vi "PLC Queue Ref Holder.vi"(6 "Action":enum16{"GET", "SET"}(ring), 8 "error in":errorcluster, 11 "Message Queue In":refnum<queue>) -> (0 "error out":errorcluster, 3 "Input Message Queue":refnum<queue>)   [LabVIEW 2015, in "PLC.lvlib"]
uses:
  PLC.lvlib
  support/Message Queue/Message Cluster.ctl
  support/Message Queue/Message Queue.lvlib
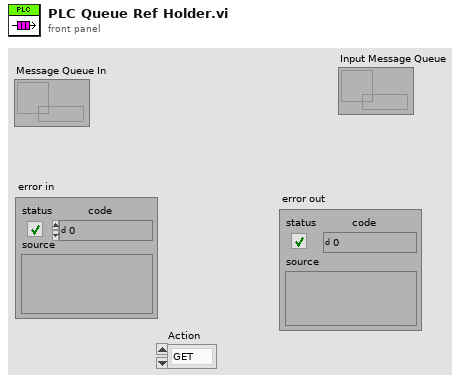
[diagram p1: front panel]
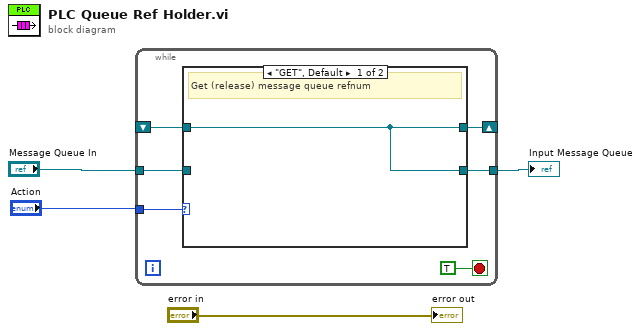
[diagram p0: block diagram]
diagram:
  n1 = while {
    shift-right: [w9] -> _
    shift-left: _ -> [w6]
    tunnel: "Message Queue In" -> [w8]
    tunnel: [w7] -> w3
    tunnel: "Action" -> [w5]
    stop <- TRUE stop-if-true
    n2 = case shown="\"GET\", Default" w5 {
      tunnel: [w11 w12] -> w9
      tunnel: w8 -> [_ w12]
      tunnel: [w11 w12] -> w7
      tunnel: w6 -> [w11 _]
      frame "GET", Default {
        # "Get (release) message queue refnum"
      }
      frame "SET" {
        # "Set (hold) message queue refnum"
      }
    }
  }
  "Input Message Queue" <- w3
  "error out" <- "error in"
